vi "SMR_LabVIEW_V3.vi"() -> ()   [LabVIEW 2025]
uses:
  <vilib>/DAQmx/read.llb/DAQmx Read (Analog 1D DBL NChan 1Samp).vi
  <vilib>/DAQmx/create/channels.llb/DAQmx Create Channel (AI-Temperature-Thermocouple).vi
  <vilib>/DAQmx/create/channels.llb/DAQmx Create Channel (AI-Voltage-Basic).vi
  <vilib>/DAQmx/miscellaneous.llb/DAQmx Fill In Error Info.vi
panel:
  out "Heat Exchanger Pressure History":dbl(graph)
  out "Main Loop Pressure History":T1(graph)
  out "Heat Exchanger Temperature History":cluster{"Waveform":dbl, "Waveform":dbl}(graph)
  out "Main Loop Temeperature History":T2(graph)
  out "Overall Avg Pressure (psi)":dbl
  out "Heat Exchanger Pressure P6 (psi)":dbl
  out "Main Loop Avg Pressure (psi)":dbl
  out "Heat Exchanger Avg Temp (deg C)":dbl
  out "Main Loop Avg Temp (deg C)":dbl
  out "Raw NI9201 \nVoltage Display":T3
  out "Temperature Display":T4
  out "Pressure Display":T5
  in  "Flow Offset Correction (GPM)":dbl=-0.3
  out "Flow History":dbl(graph)
  out "Overall Pressure History":T6(graph)
  out "Overall Temperature History":T7(graph)
  out "Max Loop Pressure (psi)":dbl
  out "Overall Avg Temp (deg C)":dbl
  out "Max Loop Temp (deg C)":dbl
  out "Heat Exchanger Flow (GPM)":dbl
  in  "Loop Period (ms)":dbl=1000.0
  in  "Stop":bool
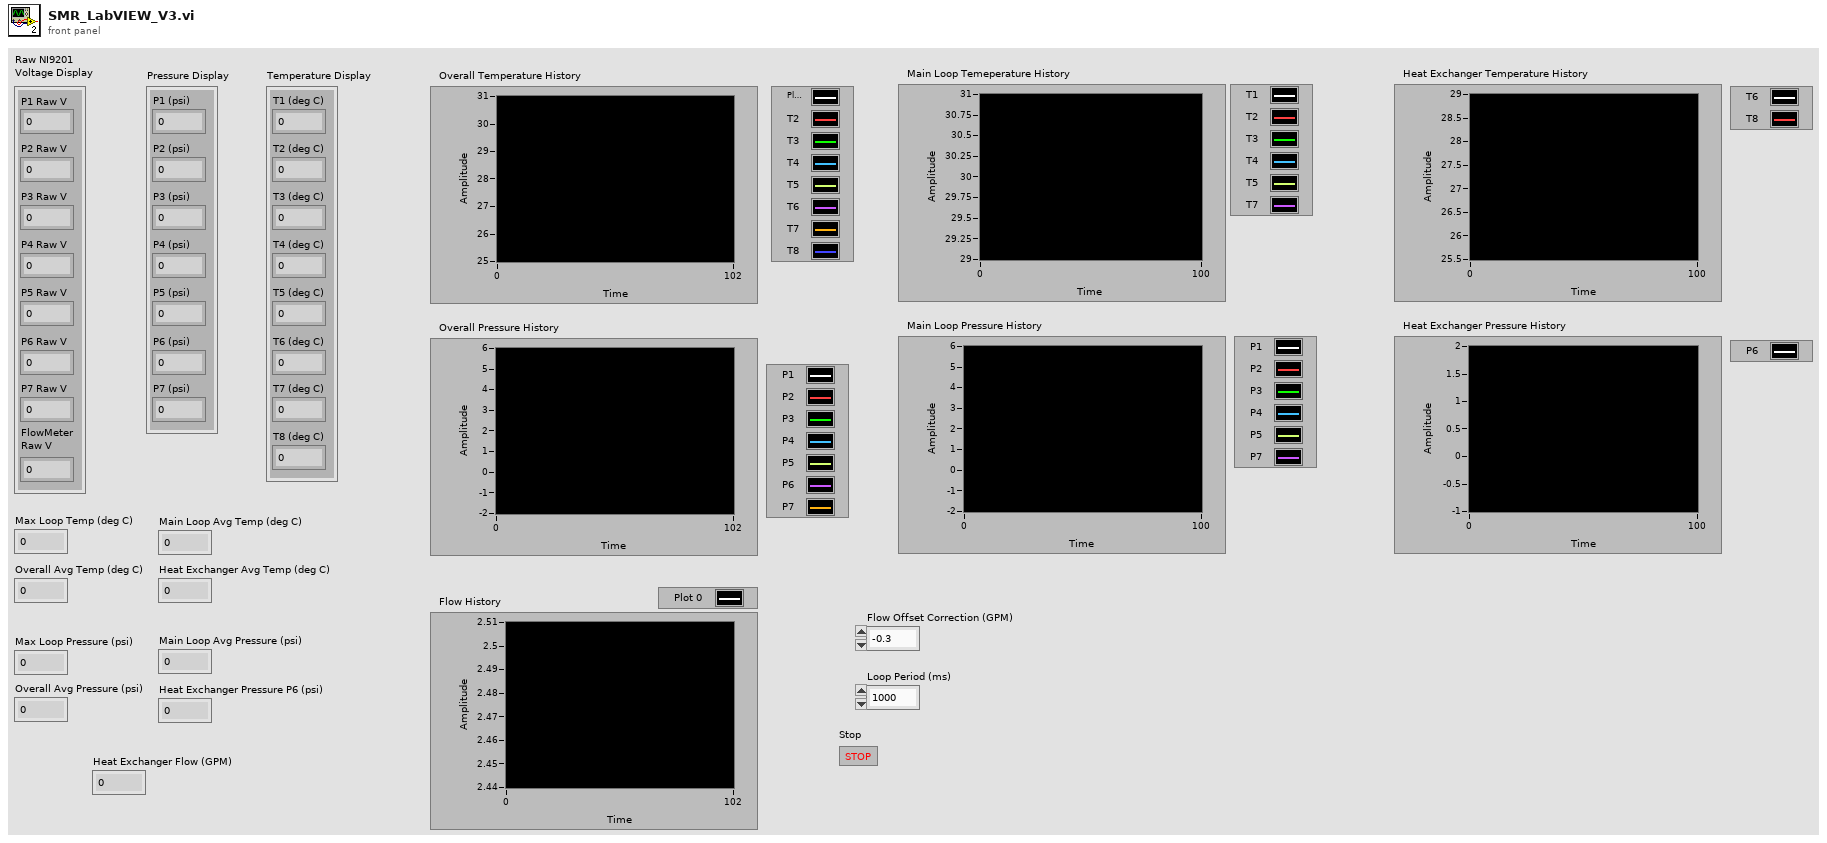
[diagram p1: front panel]
types:
  T1 = cluster{"P1":dbl, "P2":dbl, "P3":dbl, "P4":dbl, "P5":dbl, "P7":dbl}
  T2 = cluster{"Waveform":dbl, "Waveform":dbl, "Waveform":dbl, "Waveform":dbl, "Waveform":dbl, "Waveform":dbl}
  T3 = cluster{"P1 Raw V":dbl, "P2 Raw V":dbl, "P3 Raw V":dbl, "P4 Raw V":dbl, "P5 Raw V":dbl, "P6 Raw V":dbl, "P7 Raw V":dbl, "FlowMeter\nRaw V":dbl}
  T4 = cluster{"T1 (deg C)":dbl, "T2 (deg C)":dbl, "T3 (deg C)":dbl, "T4 (deg C)":dbl, "T5 (deg C)":dbl, "T6 (deg C)":dbl, "T7 (deg C)":dbl, "T8 (deg C)":dbl}
  T5 = cluster{"P1 (psi)":dbl, "P2 (psi)":dbl, "P3 (psi)":dbl, "P4 (psi)":dbl, "P5 (psi)":dbl, "P6 (psi)":dbl, "P7 (psi)":dbl}
  T6 = cluster{"P1":dbl, "P2":dbl, "P3":dbl, "P4":dbl, "P5":dbl, "P6":dbl, "P7":dbl}
  T7 = cluster{"Waveform":dbl, "Waveform":dbl, "Waveform":dbl, "Waveform":dbl, "Waveform":dbl, "Waveform":dbl, "Waveform":dbl, "Waveform":dbl}
  T8 = cluster{"P1":dbl, "P2":dbl, "P3":dbl, "P4":dbl, "P5":dbl, "P6":dbl, "P7":dbl, "Flow":dbl}
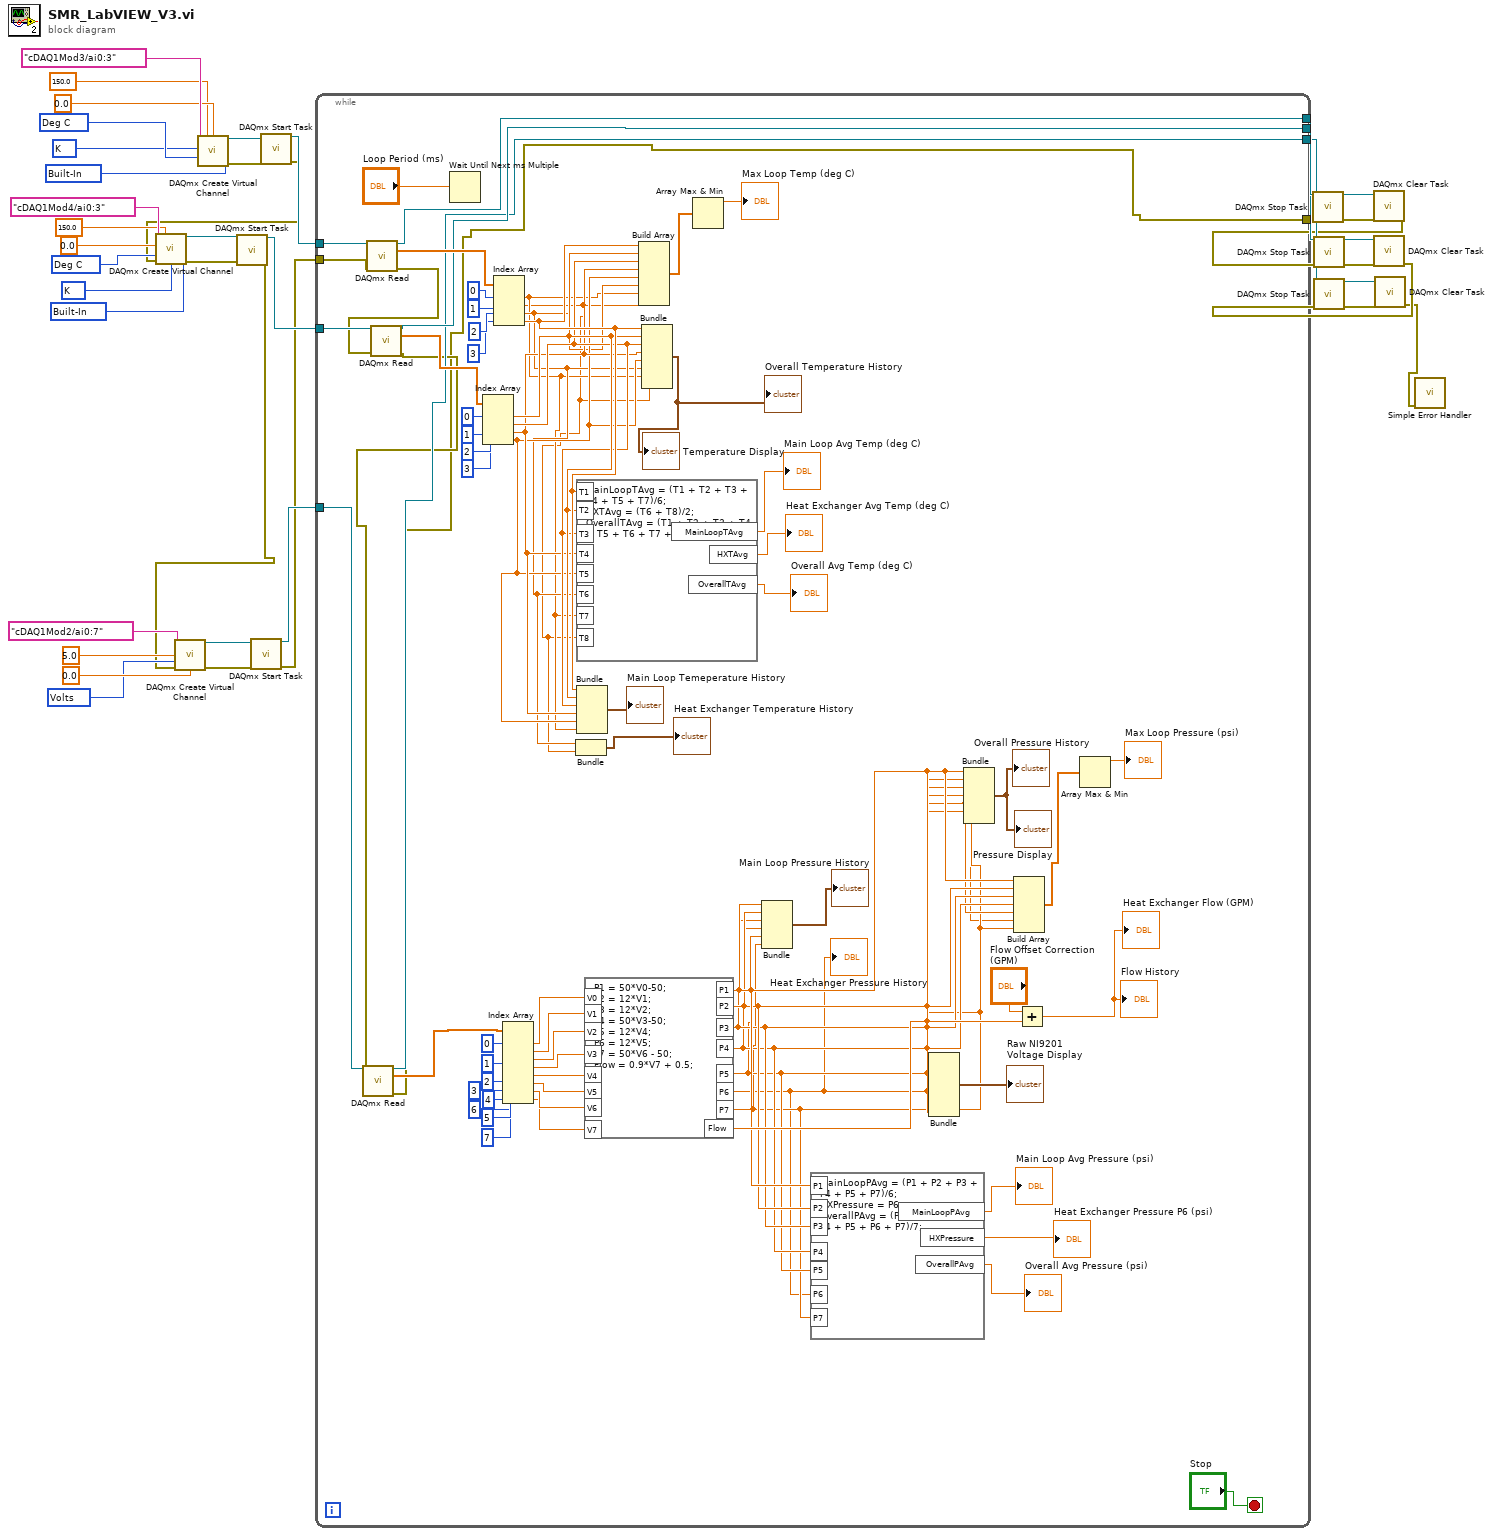
[diagram p0: block diagram]
diagram:
  w23 = 10348 items=["Volts"=10348, "From Custom Scale"=10065] ("units")
  w27 = 10200 items=["Built-In"=10200, "Constant Value"=10116, "Channel"=10113] ("cjc source")
  w28 = 10073 items=["J"=10072, "K"=10073, "N"=10077, "R"=10082, "S"=10085, "T"=10086, "B"=10047, "E"=10055] ("thermocouple type")
  w11 = 10143 items=["Deg C"=10143, "Deg F"=10144, "Kelvins"=10325, "Deg R"=10145, "From Custom Scale"=10065] ("units")
  w31 = 10200 items=["Built-In"=10200, "Constant Value"=10116, "Channel"=10113] ("cjc source")
  w32 = 10073 items=["J"=10072, "K"=10073, "N"=10077, "R"=10082, "S"=10085, "T"=10086, "B"=10047, "E"=10055] ("thermocouple type")
  w35 = 10143 items=["Deg C"=10143, "Deg F"=10144, "Kelvins"=10325, "Deg R"=10145, "From Custom Scale"=10065] ("units")
  n1 = call-poly <vilib>:"DAQmx Create Virtual Channel.vi"("maximum value"=150.0, "minimum value"=0.0, "physical channels"=tag "cDAQ1Mod3/ai0:3", "cjc source"=w31, "units"=w35, "thermocouple type"=w32) -> ("task out"=w40:refnum<k21>, "error out"=w39:errorcluster)  [unwired: 8 in]
  n2 = call <vilib>:"DAQmx Start Task.vi"("task/channels in"=w40, "error in"=w39) -> ("task out"=w20:refnum<k21>, "error out"=w10:errorcluster)  [unwired: 12 in]
  n3 = call-poly <vilib>:"DAQmx Create Virtual Channel.vi"("maximum value"=150.0, "minimum value"=0.0, "physical channels"=tag "cDAQ1Mod4/ai0:3", "cjc source"=w27, "units"=w11, "error in"=w10, "thermocouple type"=w28) -> ("task out"=w37:refnum<k21>, "error out"=w36:errorcluster)  [unwired: 7 in]
  n4 = call <vilib>:"DAQmx Start Task.vi"("task/channels in"=w37, "error in"=w36) -> ("task out"=w19:refnum<k21>, "error out"=w9:errorcluster)  [unwired: 12 in]
  n5 = call-poly <vilib>:"DAQmx Create Virtual Channel.vi"("maximum value"=5.0, "minimum value"=0.0, "physical channels"=tag "cDAQ1Mod2/ai0:7", "units"=w23, "error in"=w9) -> ("task out"=w22:refnum<k21>, "error out"=w21:errorcluster)  [unwired: 9 in]
  n6 = call <vilib>:"DAQmx Start Task.vi"("task/channels in"=w22, "error in"=w21) -> ("task out"=w18:refnum<k21>, "error out"=w8:errorcluster)  [unwired: 12 in]
  n7 = while {
    tunnel: w20 -> [w112]
    tunnel: w19 -> [w111]
    tunnel: w18 -> [w98]
    tunnel: [w79] -> w17
    tunnel: [w78] -> w16
    tunnel: [w77] -> w15
    tunnel: w8 -> [w76]
    tunnel: [w73] -> w7
    stop <- "Stop" stop-if-true
    n8 = call-poly <vilib>:"DAQmx Read.vi"("task/channels in"=w112, "error in"=w76) -> ("task out"=w79:refnum<k21>, "data"=w102:dbl[], "error out"=w75:errorcluster)  [unwired: 11 in]
    n9 = call-poly <vilib>:"DAQmx Read.vi"("task/channels in"=w111, "error in"=w75) -> ("task out"=w78:refnum<k21>, "data"=w101:dbl[], "error out"=w74:errorcluster)  [unwired: 11 in]
    n10 = call-poly <vilib>:"DAQmx Read.vi"("task/channels in"=w98, "error in"=w74) -> ("task out"=w77:refnum<k21>, "data"=w89:dbl[], "error out"=w73:errorcluster)  [unwired: 11 in]
    n11 = Wait Until Next ms Multiple(millisecond multiple="Loop Period (ms)") -> ()  [unwired: 1 out]
    n12 = Index Array(array=w101, index #1=0 ("index"), index #2=1 ("index"), index #3=2 ("index"), index #4=3 ("index")) -> (element #1=w58:dbl, element #2=w57:dbl, element #3=w56:dbl, element #4=w55:dbl)
    n13 = Index Array(array=w102, index #1=0 ("index"), index #2=1 ("index"), index #3=2 ("index"), index #4=3 ("index")) -> (element #1=w52:dbl, element #2=w51:dbl, element #3=w53:dbl, element #4=w59:dbl)
    n14 = Index Array(array=w89, index #1=0 ("index"), index #2=1 ("index"), index #3=2 ("index"), index #4=3 ("index"), index #5=4 ("index"), index #6=5 ("index"), index #7=6 ("index"), index #8=7 ("index")) -> (element #1=w88:dbl, element #2=w87:dbl, element #3=w86:dbl, element #4=w85:dbl, element #5=w84:dbl, element #6=w83:dbl, element #7=w82:dbl, element #8=w81:dbl)
    n15 = Bundle("Waveform"=w53, "Waveform"=w51) -> (→"Heat Exchanger Temperature History":cluster{"Waveform":dbl, "Waveform":dbl})  [unwired: 1 in]
    n16 = formula code="MainLoopTAvg = (T1 + T2 + T3 + T4 + T5 + T7)/6;\nHXTAvg = (T6 + T8)/2;\nOverallTAvg = (T1 + T2 + T3 + T4 + T5 + T6 + T7 + T8)/8;"("T1"=w59, "T2"=w58, "T3"=w57, "T4"=w56, "T5"=w55, "T6"=w53, "T7"=w52, "T8"=w51) -> ("MainLoopTAvg"=→"Main Loop Avg Temp (deg C)":dbl, "HXTAvg"=→"Heat Exchanger Avg Temp (deg C)":dbl, "OverallTAvg"=→"Overall Avg Temp (deg C)":dbl)
    n17 = Bundle("Waveform"=w59, "Waveform"=w58, "Waveform"=w57, "Waveform"=w56, "Waveform"=w55, "Waveform"=w52) -> (→"Main Loop Temeperature History":T2)  [unwired: 1 in]
    n18 = formula code="P1 = 50*V0-50;\nP2 = 12*V1;\nP3 = 12*V2;\nP4 = 50*V3-50;\nP5 = 12*V4;\nP6 = 12*V5; \nP7 = 50*V6 - 50;\nFlow = 0.9*V7 + 0.5;"("V0"=w88, "V1"=w87, "V2"=w86, "V3"=w85, "V4"=w84, "V5"=w83, "V6"=w82, "V7"=w81) -> ("P1"=w49:dbl, "P2"=w48:dbl, "P3"=w47:dbl, "P4"=w46:dbl, "P5"=w45:dbl, "P6"=w42:dbl, "P7"=w44:dbl, "Flow"=w67:dbl)
    "Heat Exchanger Pressure History" <- w42
    n19 = Build Array(w59, w58, w57, w56, w55, w53, w52, w51) -> (w99:dbl[])
    n20 = Bundle("Waveform"=w59, "Waveform"=w58, "Waveform"=w57, "Waveform"=w56, "Waveform"=w55, "Waveform"=w53, "Waveform"=w52, "Waveform"=w51) -> (→"Overall Temperature History" →"Temperature Display":T7)  [unwired: 1 in]
    n21 = Array Max & Min(array=w99) -> (max value=→"Max Loop Temp (deg C)":dbl)  [unwired: 3 out]
    n22 = Bundle("P1"=w49, "P2"=w48, "P3"=w47, "P4"=w46, "P5"=w45, "P7"=w44) -> (→"Main Loop Pressure History":T1)  [unwired: 1 in]
    n23 = formula code="MainLoopPAvg = (P1 + P2 + P3 + P4 + P5 + P7)/6;\nHXPressure = P6;\nOverallPAvg = (P1 + P2 + P3 + P4 + P5 + P6 + P7)/7;"("P1"=w49, "P2"=w48, "P3"=w47, "P4"=w46, "P5"=w45, "P6"=w42, "P7"=w44) -> ("MainLoopPAvg"=→"Main Loop Avg Pressure (psi)":dbl, "HXPressure"=→"Heat Exchanger Pressure P6 (psi)":dbl, "OverallPAvg"=→"Overall Avg Pressure (psi)":dbl)
    n24 = Bundle("P1"=w49, "P2"=w48, "P3"=w47, "P4"=w46, "P5"=w45, "P6"=w42, "P7"=w44, "Flow"=w67) -> (→"Raw NI9201 \nVoltage Display":T8)  [unwired: 1 in]
    n25 = Bundle("P1"=w49, "P2"=w48, "P3"=w47, "P4"=w46, "P5"=w45, "P6"=w42, "P7"=w44) -> (→"Overall Pressure History" →"Pressure Display":T6)  [unwired: 1 in]
    n26 = Build Array(w49, w48, w47, w46, w45, w42, w44) -> (w70:dbl[])
    n27 = Add(x="Flow Offset Correction (GPM)", y=w67) -> (x+y=→"Heat Exchanger Flow (GPM)" →"Flow History":dbl)
    n28 = Array Max & Min(array=w70) -> (max value=→"Max Loop Pressure (psi)":dbl)  [unwired: 3 out]
  }
  n29 = call <vilib>:"DAQmx Stop Task.vi"("task/channels in"=w17, "error in"=w7) -> ("task out"=w14:refnum<k21>, "error out"=w6:errorcluster)  [unwired: 12 in]
  n30 = call <vilib>:"DAQmx Clear Task.vi"("task in"=w14, "error in"=w6) -> ("error out"=w5:errorcluster)  [unwired: 13 in]
  n31 = call <vilib>:"DAQmx Stop Task.vi"("task/channels in"=w16, "error in"=w5) -> ("task out"=w13:refnum<k21>, "error out"=w4:errorcluster)  [unwired: 12 in]
  n32 = call <vilib>:"DAQmx Clear Task.vi"("task in"=w13, "error in"=w4) -> ("error out"=w3:errorcluster)  [unwired: 13 in]
  n33 = call <vilib>:"DAQmx Stop Task.vi"("task/channels in"=w15, "error in"=w3) -> ("task out"=w12:refnum<k21>, "error out"=w2:errorcluster)  [unwired: 12 in]
  n34 = call <vilib>:"DAQmx Clear Task.vi"("task in"=w12, "error in"=w2) -> ("error out"=w1:errorcluster)  [unwired: 13 in]
  n35 = call <vilib>:"Simple Error Handler.vi"("error in (no error)"=w1) -> ()  [unwired: 4 in, 5 out]
